vi "Write Multiple Coils Request.vi"(8 "error in (no error)":errorcluster, 9 "coils to write":bool[](array[boolean]), 10 "starting address":u16) -> (0 "error out":errorcluster, 2 "Modbus data unit out":refnum<class "Modbus Data Unit (PDU).lvclass">)   [LabVIEW 2020, in "SubVIs.lvlib" / "Master Function Definition.lvlib"]
doc: "This VI forms a modbus data unit for writing multiple coils."
uses:
  <vilib>/Modbus/subvis/Data and Functions/Master Function Definition/Master Function Definition.lvlib
  <vilib>/Modbus/subvis/Modbus Data Unit (PDU)/Modbus Data Unit (PDU).lvclass
  <vilib>/Modbus/subvis/Modbus Data Unit (PDU)/Modbus Data Unit (PDU).lvclass/Modbus Data Unit (PDU).ctl
  <vilib>/Modbus/subvis/SubVIs.lvlib
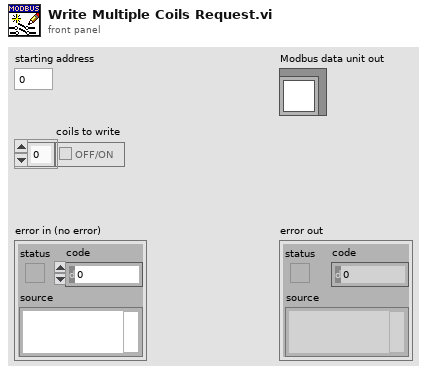
[diagram p1: front panel]
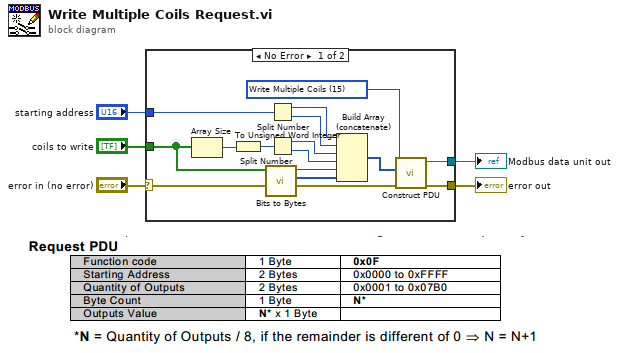
[diagram p0: block diagram]
diagram:
  n1 = case shown="No Error" "error in (no error)" {
    selector: "error in (no error)" -> [w6 w21]
    tunnel: [w20 w21] -> w5
    tunnel: "starting address" -> [w19 _]
    tunnel: [w18 _] -> w3
    tunnel: "coils to write" -> [w10 _]
    frame No Error {
      w13 = u8 15 items=["Read Discrete Inputs"=2, "Read Coils"=1, "Write Single Coil"=5, "Write Multiple Coils"=15, "Read Input Register"=4, "Read Holding Registers"=3, "Write Single Register"=6, "Write Multiple Registers"=16, "Read/Write Multiple Registers"=23, "Mask Write Register"=22, "Read FIFO Queue"=24, "Read File Record"=20, "Write File Record"=21, "Read Exception Status"=7, "Diagnostic"=8, "Get Com Event Counter"=11, "Get Com Event Log"=12, "Report Slave ID"=17, "Read Device Identification"=43] ("Function")
      n2 = Array Size(array=w10) -> (size(s)=w12:i32)
      n3 = To Unsigned Word Integer(number=w12) -> (unsigned 16bit integer=w11:u16)
      n4 = call <vilib>:"Bits to Bytes.vi"("bits"=w10) -> ("bytes"=w8:u8[], "count"=w9:u8)  [unwired: 9 in]
      n5 = Split Number(x=w19) -> (hi(x)=w14:u8, lo(x)=w15:u8)
      n6 = Split Number(x=w11) -> (hi(x)=w16:u8, lo(x)=w17:u8)
      n7 = Build Array (concatenate)(w14, w15, w16, w17, w9, w8) -> (w7:u8[])
      n8 = call <vilib>:"Construct PDU.vi"("error in (no error)"=w6, "data"=w7, "function"=w13) -> ("error out"=w20:errorcluster, "Modbus data unit out"=w18:refnum<class "Modbus Data Unit (PDU).lvclass">)  [unwired: 7 in]
    }
    frame Error {
    }
  }
  "error out" <- w5
  "Modbus data unit out" <- w3
